vi "CubeLayerGen.vi"(6 "Layer":u32=160, 10 "HatchPow":T5={"Power"=300.0, "Mark Speed"=400.0, "Jump Speed"=1000.0, "JumpPower"=0.0}, 11 "RectHatch":T6={"Width"=10.0, "Height"=10.0, "Angle"=45.0, "OffX"=0.1, "OffY"=0.1, "Spacing"=0.1, "IslandSize"=0.1} {"IslandSize" format="%#_13g"; "Spacing" format="%#_13g"; "OffY" format="%#_13g"; "OffX" format="%#_13g"; "Height" format="%#_13g"; "Width" format="%#_13g"}) -> (3 "PathSups":T1[](array[typedef]))   [LabVIEW 2014]
uses:
  TypeDefs/RectHatch.ctl
  TypeDefs/PowerSpeed.ctl
  TypeDefs/PathSupreme.ctl
  PSup2SCAN/Sub/VelocityProfile.ctl
  PSup2SCAN/Sub/PathCut.ctl
  PSup2SCAN/Sub/Segment.ctl
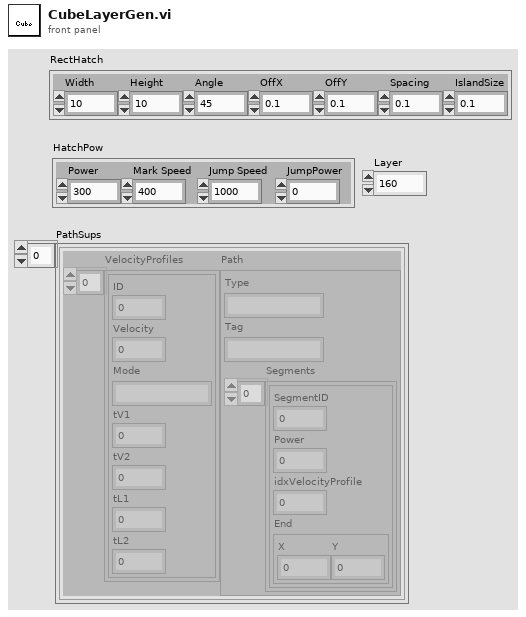
[diagram p1: front panel]
types:
  T1 = typedef "PathSupreme.ctl" = cluster{"VelocityProfiles":T2[], "Path":T3}
  T2 = typedef "VelocityProfile.ctl" = cluster{"ID":u32, "Velocity":dbl, "Mode":string, "tV1":u32, "tV2":u32, "tL1":u32, "tL2":u32}
  T3 = typedef "PathCut.ctl" = cluster{"Type":string, "Tag":string, "Segments":T4[]}
  T4 = typedef "Segment.ctl" = cluster{"SegmentID":u16, "Power":sgl, "idxVelocityProfile":u16, "End":cluster{"X":sgl, "Y":sgl}}
  T5 = typedef "PowerSpeed.ctl" = cluster{"Power":dbl, "Mark Speed":dbl, "Jump Speed":dbl, "JumpPower":dbl}
  T6 = typedef "RectHatch.ctl" = cluster{"Width":dbl, "Height":dbl, "Angle":sgl, "OffX":dbl, "OffY":dbl, "Spacing":dbl, "IslandSize":dbl}
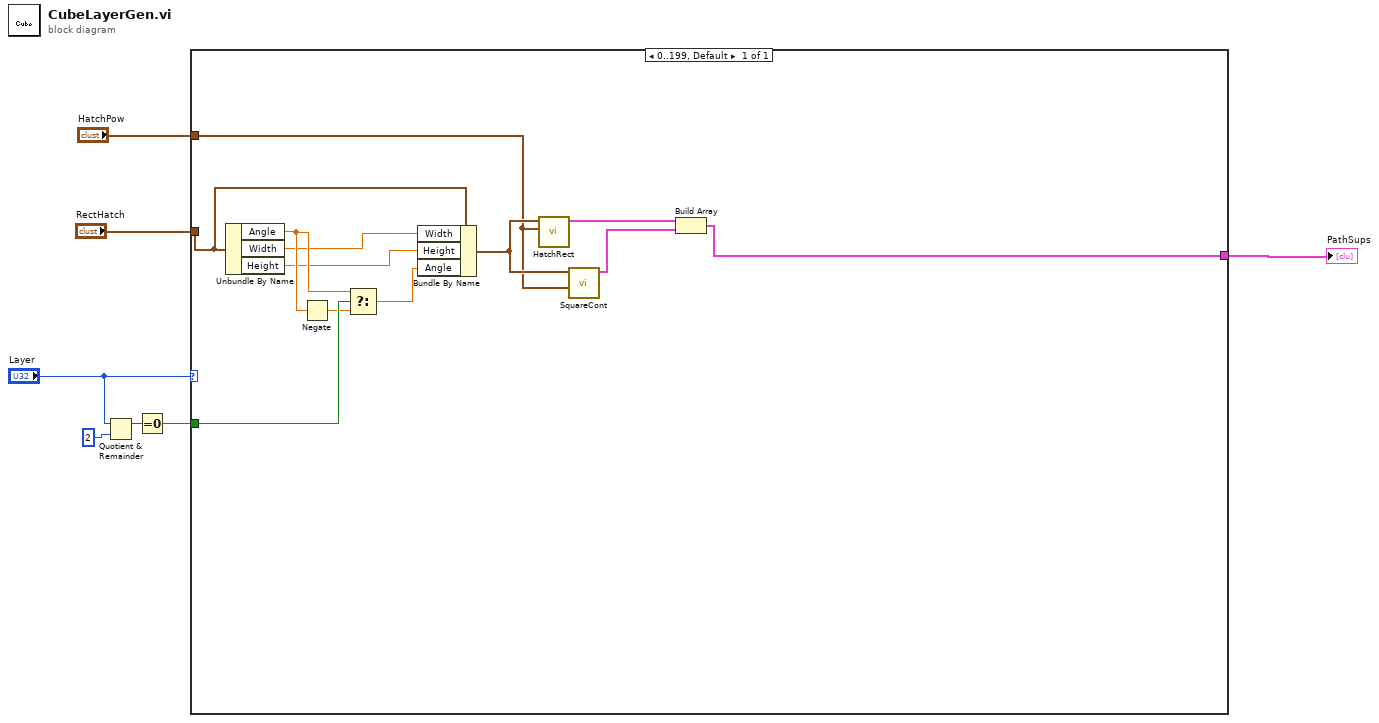
[diagram p0: block diagram]
diagram:
  n1 = Quotient & Remainder(x="Layer", y=u8 2) -> (x-y*floor(x/y)=w7:u32)  [unwired: 1 out]
  n2 = Equal To 0?(x=w7) -> (x = 0?=w4:bool)
  n3 = case shown="0..199, Default" "Layer" {
    tunnel: w4 -> [w19]
    tunnel: "RectHatch" -> [w18]
    tunnel: "HatchPow" -> [w11]
    tunnel: [w12] -> w1
    frame 0..199, Default {
      n4 = Unbundle By Name(w18) -> ("Angle"=w16:sgl, "Width"=w9:dbl, "Height"=w8:dbl)
      n5 = Negate(x=w16) -> (-x=w17:sgl)
      n6 = Select(t=w16, s=w19, f=w17) -> (s? t:f=w15:sgl)
      n7 = Bundle By Name(cluster=w18, "Width"=w9, "Height"=w8, "Angle"=w15) -> (w14:T6)
      n8 = call "HatchRect.vi"("HatchPow"=w11, "RectHatch"=w14) -> ("PathSupreme"=w13:T1)  [unwired: 9 in]
      n9 = call "SquareCont.vi"("ContPow"=w11, "RectHatch"=w14) -> ("PathSupreme"=w10:T1)  [unwired: 9 in]
      n10 = Build Array(w13, w10) -> (w12:T1[])
    }
  }
  "PathSups" <- w1
